vi "TestExec.Set Result State.vi"(6 "Code Enum":T1=-6100 items=["No Error"=0, "Abort"=-2, "Misc"=-5000, "Fixture Error"=-5100, "File IO - General"=-5200, "FIle IO - Config Error"=-5201, "Instrument - General"=-5300, "Instrument - Serial Com"=-5301, "Instrument - Camera"=-5302, "Instrument - PS"=-5303, "Instrument - Oscilloscope"=-5304, "Instrument - Function Gen"=-5305, "Instrument - Load"=-5306, "Instrument - Meter"=-5307, "Instrument - Power Control"=-5308, "Instrument - Motion"=-5309, "Instrument - RF"=-5310, "System Exe"=-5400, "Image Processing"=-5500, "Communication"=-5600, "Script - Syntax Error"=-6000, "Script - Invalid Name or Param"=-6100, "Script - Timeout"=-6200, "Invalid Data"=-6300, "FW Update Error"=-6500], 7 "Limits":variant, 8 "Description":string, 9 "Code Int":i32=-1, 10 "State":T3=enum."ABORT", 11 "Result State In":T2={"State"=enum."Passing", "Code"=0, "Description"=""}) -> (3 "Result State Out":T2={"State"=enum."Passing", "Code"=0, "Description"=""})   [LabVIEW 2018]
uses:
  <vilib>/KATE/SeqMgr/SeqMgr.Result State Enum.ctl
  <vilib>/KATE/SeqMgr/SeqMgr.Result Info.ctl
  Common/Utils/Errors/Error.Error Code List.ctl
  Common/Utils/Results/Limits/Result.Test Limit Item.ctl
  Common/Utils/Results/Result.Limit Type.ctl
  <vilib>/KATE/SeqMgr/SeqMgr.lvlib
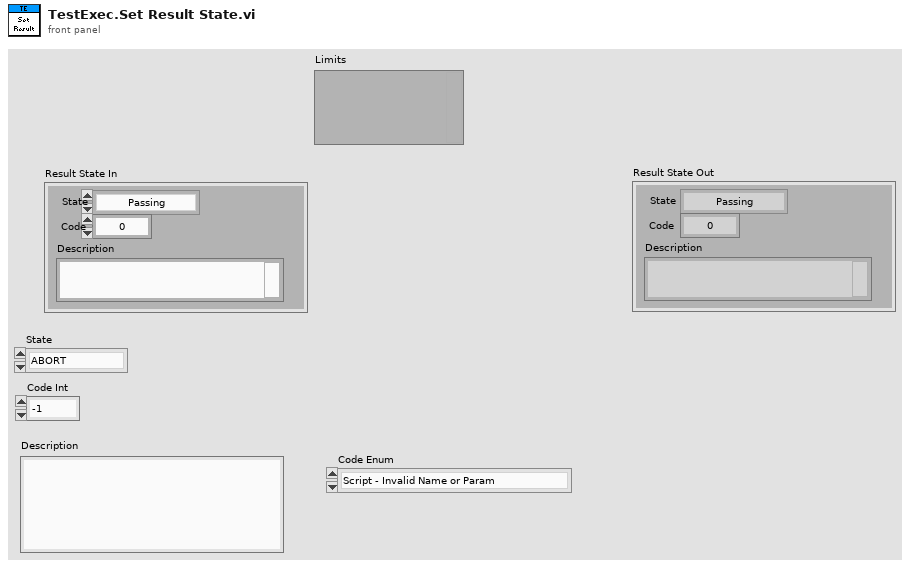
[diagram p1: front panel]
types:
  T1 = typedef "Error.Error Code List.ctl" = i32
  T2 = typedef "KATE_Lib.lvlib/SeqMgr.lvlib/SeqMgr.Result Info.ctl" = cluster{"State":T3, "Code":i32, "Description":string}
  T3 = typedef "KATE_Lib.lvlib/SeqMgr.lvlib/SeqMgr.Result State Enum.ctl" = enum16{"None", "Passing", "Failing", "PASS", "FAIL", "ABORT", "ERROR"}
  T4 = typedef "Result.Test Limit Item.ctl" = cluster{"Name":string, "LimType":T5, "LL":string, "UL":string, "Units":string, "FailCode":i32, "FailDesc":string}
  T5 = typedef "Result.Limit Type.ctl" = enum16{"None", "EQ", "NE", "GT", "LT", "GE", "LE", "GTLT", "GELE", "GELT", "GTLE", "LTGT", "LEGE", "LEGT", "LTGE", "Contains", "NotContains"}
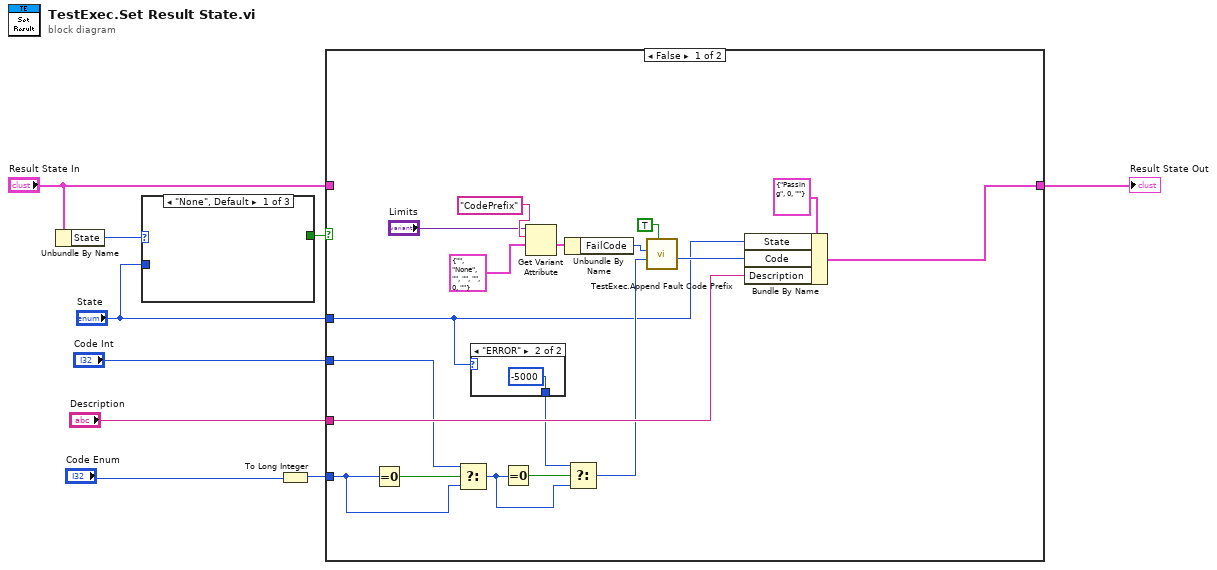
[diagram p0: block diagram]
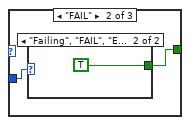
[diagram p2: hidden frame]
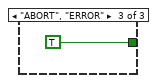
[diagram p4: hidden frame]
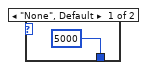
[diagram p5: hidden frame]
diagram:
  n1 = Unbundle By Name("Result State In") -> ("State"=w6:T3)
  n2 = case shown="\"None\", Default" w6 {
    tunnel: [_ w10 TRUE] -> w4
    tunnel: "State" -> [_ w11 _]
    frame "None", Default {
    }
    frame "FAIL" {
      n3 = case shown="\"Failing\", \"FAIL\", \"ERROR\"" w11 {
        tunnel: [_ TRUE] -> w10
        frame Default {
        }
        frame "Failing", "FAIL", "ERROR" {
        }
      }
    }
    frame "ABORT", "ERROR" {
    }
  }
  n4 = To Long Integer(number="Code Enum") -> (32bit integer=w2:T1)
  n5 = case shown="False" w4 {
    tunnel: "State" -> [w15 _]
    tunnel: "Code Int" -> [w17 _]
    tunnel: "Description" -> [w24 _]
    tunnel: [w22 w34] -> w7
    tunnel: "Result State In" -> [_ w34]
    tunnel: w2 -> [w20 _]
    frame False {
      n6 = Equal To 0?(x=w20) -> (x = 0?=w21:bool)
      n7 = Select(t=w17, s=w21, f=w20) -> (s? t:f=w18:T1)
      n8 = case shown="\"ERROR\"" w15 {
        tunnel: [5000 -5000] -> w14
        frame "None", Default {
        }
        frame "ERROR" {
        }
      }
      n9 = Equal To 0?(x=w18) -> (x = 0?=w19:bool)
      n10 = Get Variant Attribute(Variant="Limits", name="CodePrefix", default value (empty Variant)=T4 {"Name"="", "LimType"=enum."None", "LL"="", "UL"="", "Units"="", "FailCode"=0, "FailDesc"=""} ("Result.Test Limit Item")) -> (value=w30:T4)  [unwired: 1 in, 3 out]
      n11 = Unbundle By Name(w30) -> ("FailCode"=w27:i32)
      n12 = Select(t=w14, s=w19, f=w18) -> (s? t:f=w16:T1)
      n13 = call "TestExec.Append Fault Code Prefix.vi"("Positive(F)\\Negative(T)"=TRUE ("Positive(F)\\Negative(T)"), "FaultCode"=w16, "FaultCode Prefix"=w27) -> ("New Fault Code"=w26:i32)  [unwired: 8 in]
      n14 = Bundle By Name(cluster=T2 {"State"=enum."Passing", "Code"=0, "Description"=""} ("ResultState"), "State"=w15, "Code"=w26, "Description"=w24) -> (w22:T2)
    }
    frame True {
      # "Due nothing.  Current result is already ERROR/FAIL"
    }
  }
  "Result State Out" <- w7
